vi "Page_Info_Initialize.vi"(8 "error in (no error)":errorcluster, 9 "ctlReferences":T1, 11 "AB_WebService in":refnum<class "AB_WebService.lvclass">) -> (0 "error out":errorcluster, 3 "AB_WebService out":refnum<class "AB_WebService.lvclass">)   [LabVIEW 2020, in "AB_WebService.lvclass"]
uses:
  <vilib>/AppBuilder/AB_Classes/WebService/AB_WebService.lvclass
  <resource>/Framework/Providers/Builds/AppBuilder/AB_UI_Page_Info_References.ctl
  <resource>/Framework/Providers/Common/provcom_StringGlobals.vi
  <vilib>/AppBuilder/AB_Classes/TargetFile/AB_Targetfile.lvclass
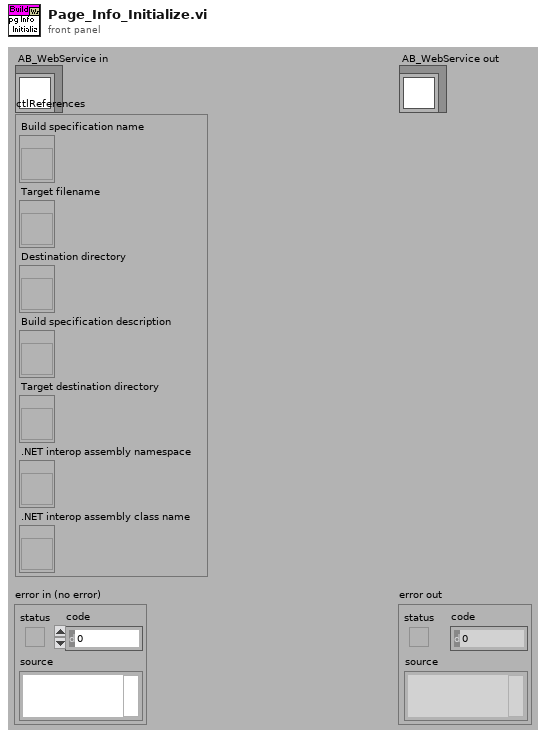
[diagram p1: front panel]
types:
  T1 = typedef "AB_UI_Page_Info_References.ctl" = cluster{"Build specification name":refnum<vi>, "Target filename":refnum<vi>, "Destination directory":refnum<vi>, "Build specification description":refnum<vi>, "Target destination directory":refnum<vi>, ".NET interop assembly namespace":refnum<vi>, ".NET interop assembly class name":refnum<vi>}
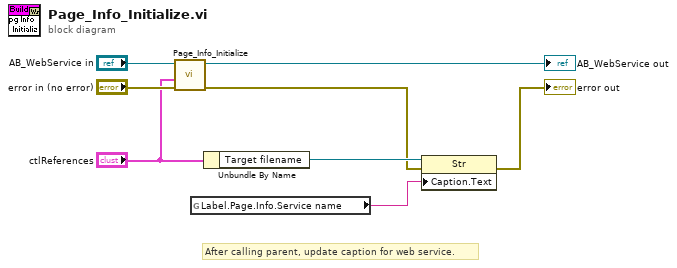
[diagram p0: block diagram]
diagram:
  # "After calling parent, update caption for web service."
  n1 = call-parent "Page_Info_Initialize.vi"("error in (no error)"="error in (no error)", "ctlReferences"="ctlReferences", "AB_Targetfile in"="AB_WebService in") -> ("error out"=w3:errorcluster, "AB_Targetfile out"=→"AB_WebService out":refnum<class "AB_WebService.lvclass">)  [unwired: 7 in]
  n2 = global read "provcom_StringGlobals.vi" "Label.Page.Info.Service name"() -> (w7:string)
  n3 = Unbundle By Name("ctlReferences") -> ("Target filename"=w8:refnum<vi>)
  n4 = property class="Str"(reference=w8, error in=w3, "Caption.Text"=w7) -> (error out=→"error out":errorcluster)  [unwired: 1 out]
